vi "首页.vi"() -> ()   [LabVIEW 2016]
uses:
  <vilib>/Utility/miscctls.llb/LVPointTypeDef.ctl
  <vilib>/addons/database/_DB Variant To Data/Database Variant To Data.xnode
  PLC/PLC.lvlib
panel:
  out "大项目框 12":T1(xcontrol)
  out "大项目框 11":T1(xcontrol)
  out "大项目框 10":T1(xcontrol)
  out "大项目框 9":T1(xcontrol)
  out "大项目框 8":T1(xcontrol)
  out "大项目框 7":T1(xcontrol)
  out "大项目框 6":T1(xcontrol)
  out "大项目框 5":T1(xcontrol)
  out "大项目框 4":T1(xcontrol)
  out "大项目框 3":T1(xcontrol)
  out "大项目框 2":T1(xcontrol)
  out "大项目框":T1(xcontrol)
  out "湿度":string="75.5 %"
  out "室温":string="25.8 ℃"
  # "室温:"
  # "湿度:"
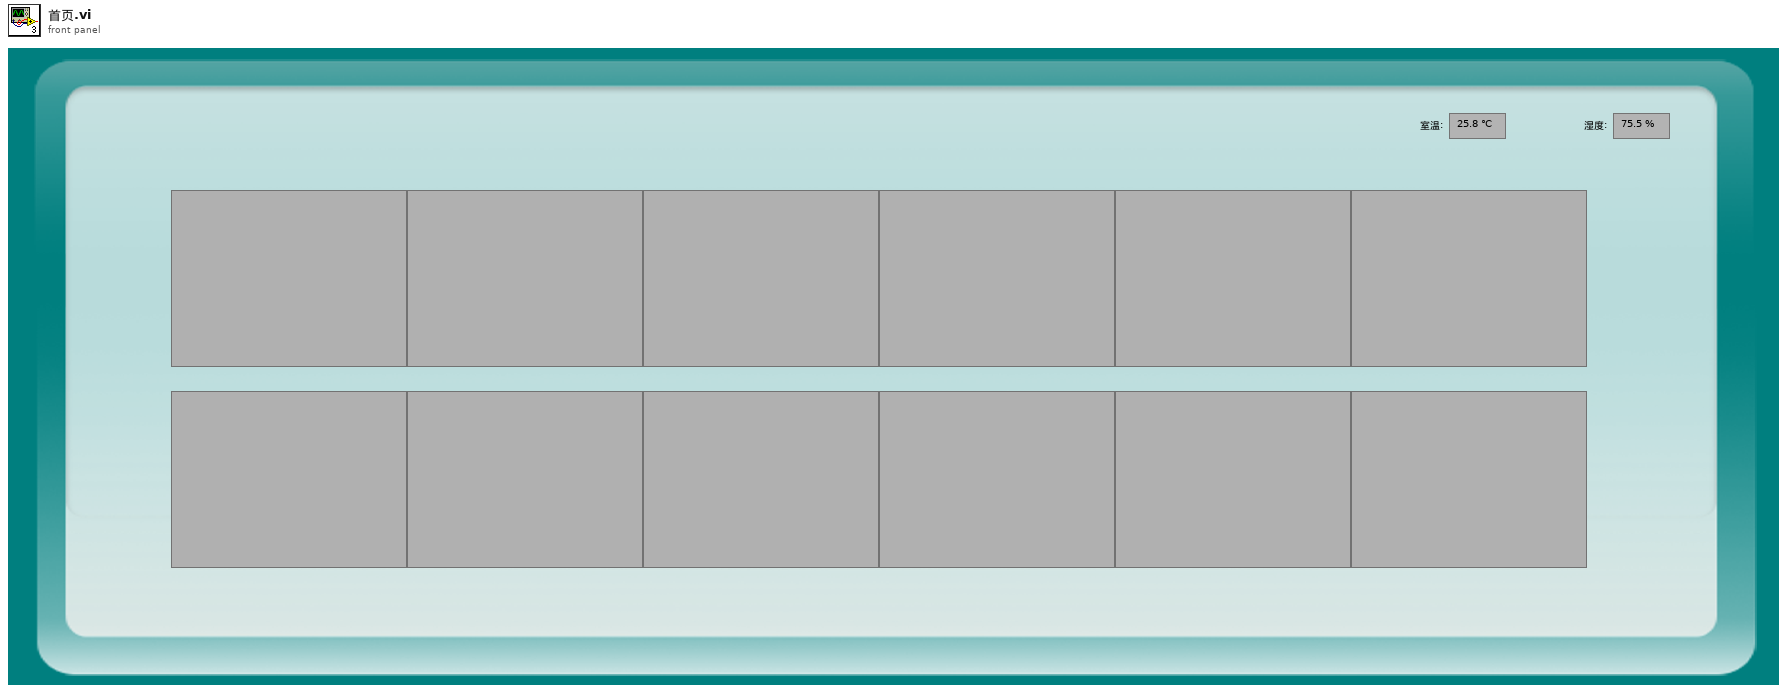
[diagram p1: front panel]
types:
  T1 = cluster{"中文项目名称":string, "英文项目名称":string, "单位":string, "浓度值":string}
  T2 = typedef "LVPointTypeDef.ctl" = cluster{"Horizontal":i16, "Vertical":i16}
  T3 = cluster{"显示参数中文名":string, "显示参数英文名":string, "显示浓度":string, "显示单位":string}[]
  T4 = cluster{"显示参数中文名":string, "显示参数英文名":string, "显示浓度":string, "显示单位":string}
  T5 = cluster{"AD0":sgl, "AD1":sgl, "AD2":sgl, "AD3":sgl, "AD4":sgl, "AD5":sgl}
  T6 = typedef "LVDateTimeRec.ctl" = cluster{"秒数的小数部分":dbl, "秒":i32, "分":i32, "时":i32, "日":i32, "月":i32, "年":i32, "天数（周）":i32, "天数（年）":i32, "DST":i32}
  T7 = cluster{"时间标识":timestamp, "监测值":sgl, "单位":string}
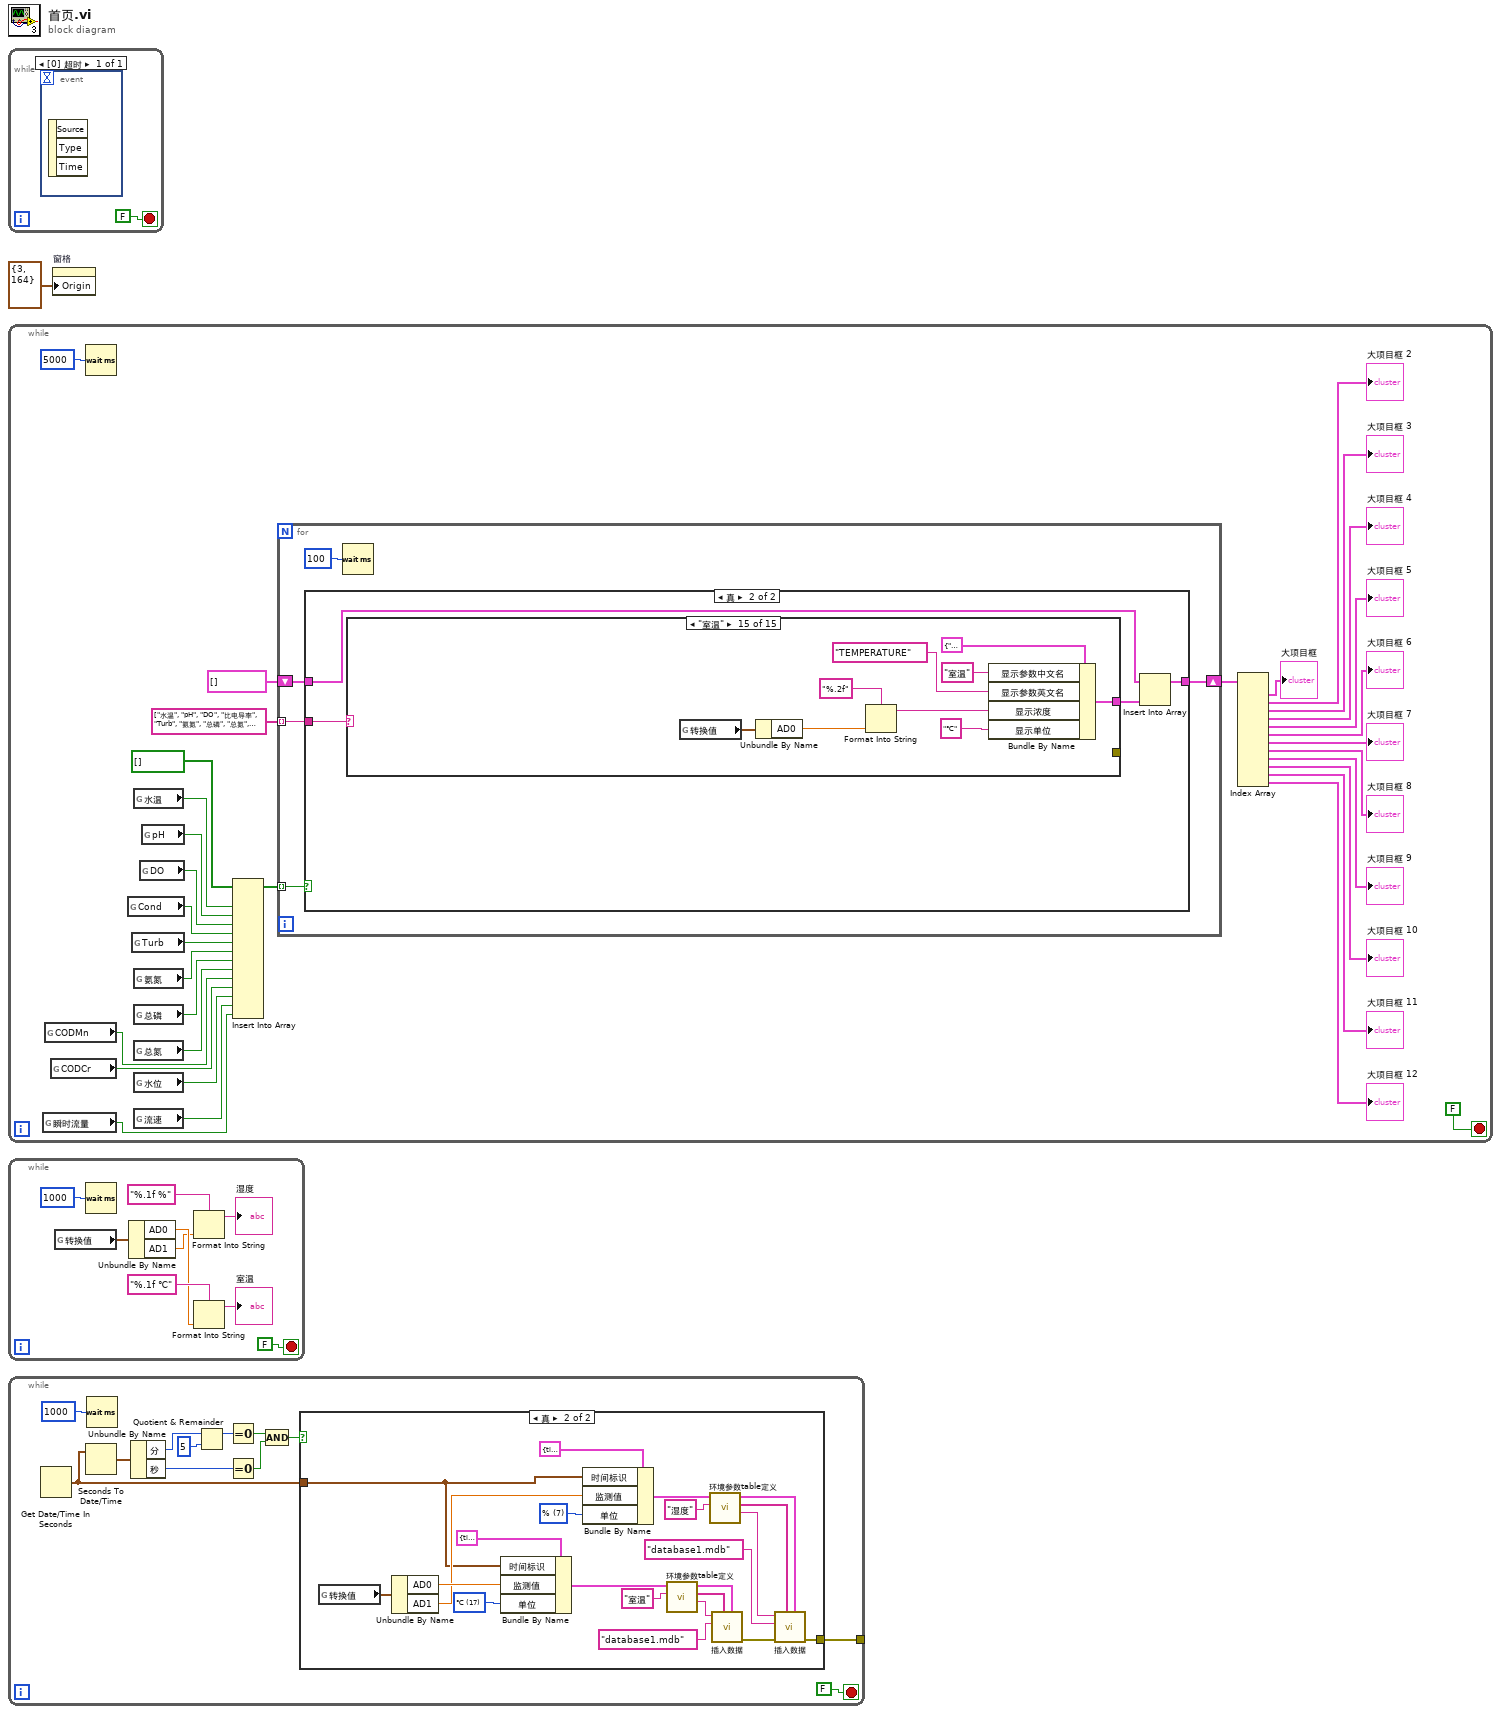
[diagram p0: block diagram]
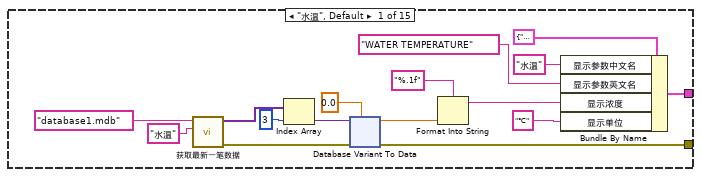
[diagram p4: hidden frame]
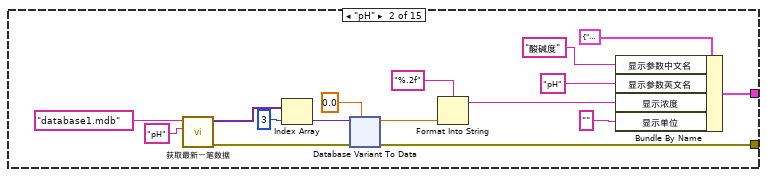
[diagram p5: hidden frame]
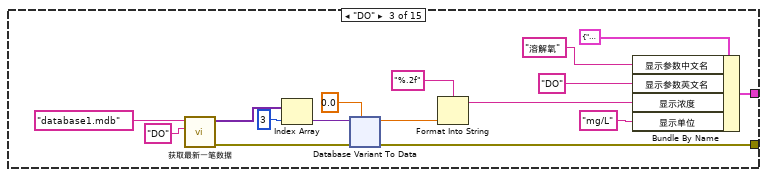
[diagram p6: hidden frame]
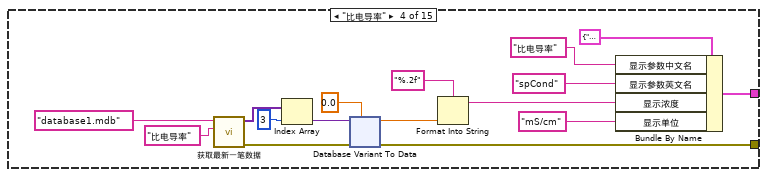
[diagram p7: hidden frame]
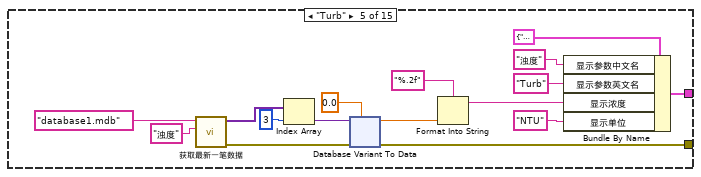
[diagram p8: hidden frame]
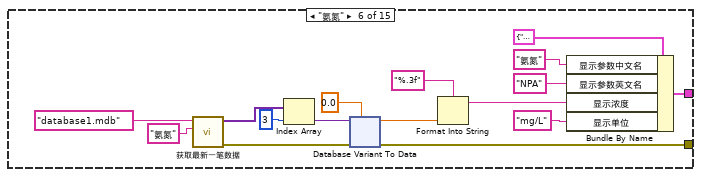
[diagram p9: hidden frame]
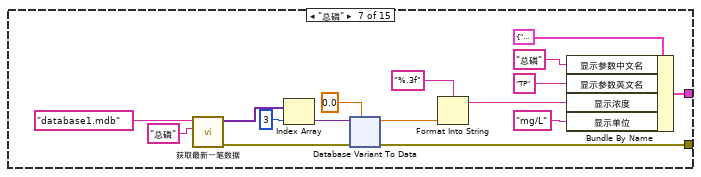
[diagram p10: hidden frame]
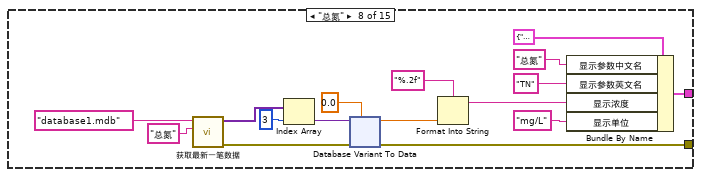
[diagram p11: hidden frame]
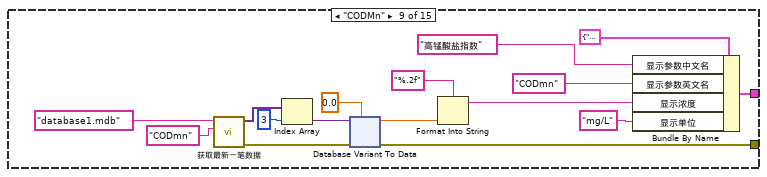
[diagram p12: hidden frame]
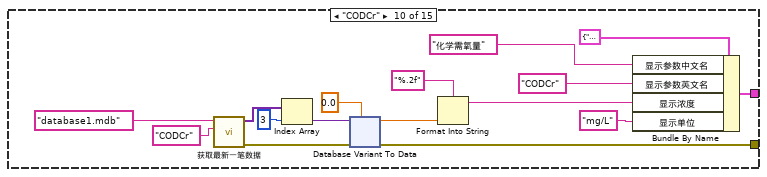
[diagram p13: hidden frame]
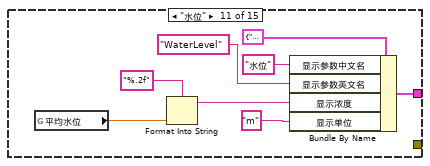
[diagram p14: hidden frame]
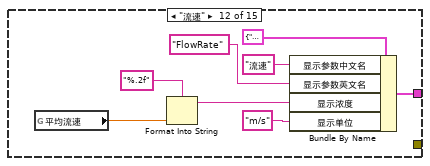
[diagram p15: hidden frame]
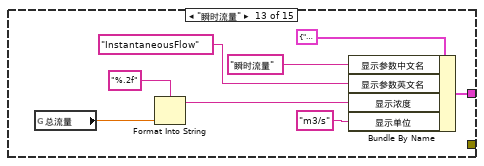
[diagram p16: hidden frame]
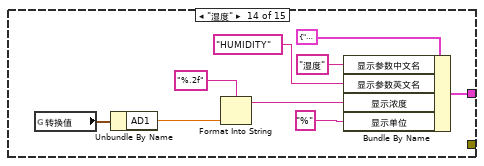
[diagram p17: hidden frame]
diagram:
  n1 = while {
    stop <- FALSE stop-if-true
    n2 = event shown="[0] 超时" {
      selector: _ -> [_]
      dyn-events: _ -> [_]
      timeout: _ -> [_]
      event Timeout {
        n3 = event-data() -> ()  [unwired: 1 in, 3 out]
      }
    }
  }
  n4 = while {
    stop <- FALSE stop-if-true
    n5 = global read "副屏设置全局变量.vi" "瞬时流量"() -> (w30:bool)
    n6 = global read "副屏设置全局变量.vi" "CODMn"() -> (w26:bool)
    n7 = global read "副屏设置全局变量.vi" "CODCr"() -> (w27:bool)
    n8 = Wait (ms)(milliseconds to wait=u32 5000 ("等待时间（毫秒）")) -> ()  [unwired: 1 out]
    n9 = global read "副屏设置全局变量.vi" "Cond"() -> (w21:bool)
    n10 = global read "副屏设置全局变量.vi" "Turb"() -> (w22:bool)
    n11 = global read "副屏设置全局变量.vi" "水温"() -> (w18:bool)
    n12 = global read "副屏设置全局变量.vi" "氨氮"() -> (w23:bool)
    n13 = global read "副屏设置全局变量.vi" "总磷"() -> (w24:bool)
    n14 = global read "副屏设置全局变量.vi" "总氮"() -> (w25:bool)
    n15 = global read "副屏设置全局变量.vi" "水位"() -> (w28:bool)
    n16 = global read "副屏设置全局变量.vi" "流速"() -> (w29:bool)
    n17 = global read "副屏设置全局变量.vi" "DO"() -> (w20:bool)
    n18 = global read "副屏设置全局变量.vi" "pH"() -> (w19:bool)
    n19 = Insert Into Array(array=bool[] [], new element #1=w18, new element #2=w19, new element #3=w20, new element #4=w21, new element #5=w22, new element #6=w23, new element #7=w24, new element #8=w25, new element #9=w26, new element #10=w27, new element #11=w28, new element #12=w29, new element #13=w30) -> (w32:bool[])  [unwired: 1 in]
    n20 = for {
      tunnel: w32 -> [w39] mode=indexing
      tunnel: string[] ["水温", "pH", "DO", "比电导率", "Turb", "氨氮", "总磷", "总氮", "CODMn", "CODCr", "水位", "流速", "瞬时流量"] -> [w38] mode=indexing
      shift-right: [w36] -> w16
      shift-left: T3 [] -> [w37]
      n21 = case shown="真" w39 {
        tunnel: w38 -> [_ w44]
        tunnel: w37 -> [w40 w43]
        tunnel: [w40 w42] -> w36
        frame False {
        }
        frame True {
          n22 = case shown="\"室温\"" w44 {
            tunnel: [w45 w104 w152 w200 w248 w296 w344 w392 w440 w488 w528 w536 w541 w553 w562] -> w41
            tunnel: [w46 w93 w141 w189 w237 w285 w333 w381 w429 w477 _ _ _ _ _] -> _
            frame "水温", Default {
              n23 = call "获取最新一笔数据.vi"("table"="水温", "database"="database1.mdb" ("名称或相对路径")) -> ("error out"=w47:errorcluster, "子数组"=w53:variant[])  [unwired: 8 in]
              n24 = Index Array(array=w53, index=3 ("索引")) -> (element=w51:variant)
              n25 = xnode "Database Variant To Data"("database variant"=w51, "error in (no error)"=w47, "type"=0.0) -> ("data"=w48:dbl, "error out"=w46:errorcluster)
              n26 = Format Into String(format string="%.1f" ("格式字符串"), w48) -> (resulting string=w55:string)  [unwired: 2 in, 1 out]
              n27 = Bundle By Name(cluster=T4 {"显示参数中文名"="", "显示参数英文名"="", "显示浓度"="", "显示单位"=""} ("元素"), "显示参数中文名"="水温", "显示参数英文名"="WATER TEMPERATURE", "显示浓度"=w55, "显示单位"="℃") -> (w45:T4)
            }
            frame "pH" {
              n28 = call "获取最新一笔数据.vi"("table"="pH", "database"="database1.mdb" ("名称或相对路径")) -> ("error out"=w94:errorcluster, "子数组"=w100:variant[])  [unwired: 8 in]
              n29 = Index Array(array=w100, index=3 ("索引")) -> (element=w98:variant)
              n30 = xnode "Database Variant To Data"("database variant"=w98, "error in (no error)"=w94, "type"=0.0) -> ("data"=w95:dbl, "error out"=w93:errorcluster)
              n31 = Format Into String(format string="%.2f" ("格式字符串"), w95) -> (resulting string=w102:string)  [unwired: 2 in, 1 out]
              n32 = Bundle By Name(cluster=T4 {"显示参数中文名"="", "显示参数英文名"="", "显示浓度"="", "显示单位"=""} ("元素"), "显示参数中文名"="酸碱度", "显示参数英文名"="pH", "显示浓度"=w102, "显示单位"="") -> (w104:T4)
            }
            frame "DO" {
              n33 = call "获取最新一笔数据.vi"("table"="DO", "database"="database1.mdb" ("名称或相对路径")) -> ("error out"=w142:errorcluster, "子数组"=w148:variant[])  [unwired: 8 in]
              n34 = Index Array(array=w148, index=3 ("索引")) -> (element=w146:variant)
              n35 = xnode "Database Variant To Data"("database variant"=w146, "error in (no error)"=w142, "type"=0.0) -> ("data"=w143:dbl, "error out"=w141:errorcluster)
              n36 = Format Into String(format string="%.2f" ("格式字符串"), w143) -> (resulting string=w150:string)  [unwired: 2 in, 1 out]
              n37 = Bundle By Name(cluster=T4 {"显示参数中文名"="", "显示参数英文名"="", "显示浓度"="", "显示单位"=""} ("元素"), "显示参数中文名"="溶解氧", "显示参数英文名"="DO", "显示浓度"=w150, "显示单位"="mg/L") -> (w152:T4)
            }
            frame "比电导率" {
              n38 = call "获取最新一笔数据.vi"("table"="比电导率", "database"="database1.mdb" ("名称或相对路径")) -> ("error out"=w190:errorcluster, "子数组"=w196:variant[])  [unwired: 8 in]
              n39 = Index Array(array=w196, index=3 ("索引")) -> (element=w194:variant)
              n40 = xnode "Database Variant To Data"("database variant"=w194, "error in (no error)"=w190, "type"=0.0) -> ("data"=w191:dbl, "error out"=w189:errorcluster)
              n41 = Format Into String(format string="%.2f" ("格式字符串"), w191) -> (resulting string=w198:string)  [unwired: 2 in, 1 out]
              n42 = Bundle By Name(cluster=T4 {"显示参数中文名"="", "显示参数英文名"="", "显示浓度"="", "显示单位"=""} ("元素"), "显示参数中文名"="比电导率", "显示参数英文名"="spCond", "显示浓度"=w198, "显示单位"="mS/cm") -> (w200:T4)
            }
            frame "Turb" {
              n43 = call "获取最新一笔数据.vi"("table"="浊度", "database"="database1.mdb" ("名称或相对路径")) -> ("error out"=w238:errorcluster, "子数组"=w244:variant[])  [unwired: 8 in]
              n44 = Index Array(array=w244, index=3 ("索引")) -> (element=w242:variant)
              n45 = xnode "Database Variant To Data"("database variant"=w242, "error in (no error)"=w238, "type"=0.0) -> ("data"=w239:dbl, "error out"=w237:errorcluster)
              n46 = Format Into String(format string="%.2f" ("格式字符串"), w239) -> (resulting string=w246:string)  [unwired: 2 in, 1 out]
              n47 = Bundle By Name(cluster=T4 {"显示参数中文名"="", "显示参数英文名"="", "显示浓度"="", "显示单位"=""} ("元素"), "显示参数中文名"="浊度", "显示参数英文名"="Turb", "显示浓度"=w246, "显示单位"="NTU") -> (w248:T4)
            }
            frame "氨氮" {
              n48 = call "获取最新一笔数据.vi"("table"="氨氮", "database"="database1.mdb" ("名称或相对路径")) -> ("error out"=w286:errorcluster, "子数组"=w292:variant[])  [unwired: 8 in]
              n49 = Index Array(array=w292, index=3 ("索引")) -> (element=w290:variant)
              n50 = xnode "Database Variant To Data"("database variant"=w290, "error in (no error)"=w286, "type"=0.0) -> ("data"=w287:dbl, "error out"=w285:errorcluster)
              n51 = Format Into String(format string="%.3f" ("格式字符串"), w287) -> (resulting string=w294:string)  [unwired: 2 in, 1 out]
              n52 = Bundle By Name(cluster=T4 {"显示参数中文名"="", "显示参数英文名"="", "显示浓度"="", "显示单位"=""} ("元素"), "显示参数中文名"="氨氮", "显示参数英文名"="NPA", "显示浓度"=w294, "显示单位"="mg/L") -> (w296:T4)
            }
            frame "总磷" {
              n53 = call "获取最新一笔数据.vi"("table"="总磷", "database"="database1.mdb" ("名称或相对路径")) -> ("error out"=w334:errorcluster, "子数组"=w340:variant[])  [unwired: 8 in]
              n54 = Index Array(array=w340, index=3 ("索引")) -> (element=w338:variant)
              n55 = xnode "Database Variant To Data"("database variant"=w338, "error in (no error)"=w334, "type"=0.0) -> ("data"=w335:dbl, "error out"=w333:errorcluster)
              n56 = Format Into String(format string="%.3f" ("格式字符串"), w335) -> (resulting string=w342:string)  [unwired: 2 in, 1 out]
              n57 = Bundle By Name(cluster=T4 {"显示参数中文名"="", "显示参数英文名"="", "显示浓度"="", "显示单位"=""} ("元素"), "显示参数中文名"="总磷", "显示参数英文名"="TP", "显示浓度"=w342, "显示单位"="mg/L") -> (w344:T4)
            }
            frame "总氮" {
              n58 = call "获取最新一笔数据.vi"("table"="总氮", "database"="database1.mdb" ("名称或相对路径")) -> ("error out"=w382:errorcluster, "子数组"=w388:variant[])  [unwired: 8 in]
              n59 = Index Array(array=w388, index=3 ("索引")) -> (element=w386:variant)
              n60 = xnode "Database Variant To Data"("database variant"=w386, "error in (no error)"=w382, "type"=0.0) -> ("data"=w383:dbl, "error out"=w381:errorcluster)
              n61 = Format Into String(format string="%.2f" ("格式字符串"), w383) -> (resulting string=w390:string)  [unwired: 2 in, 1 out]
              n62 = Bundle By Name(cluster=T4 {"显示参数中文名"="", "显示参数英文名"="", "显示浓度"="", "显示单位"=""} ("元素"), "显示参数中文名"="总氮", "显示参数英文名"="TN", "显示浓度"=w390, "显示单位"="mg/L") -> (w392:T4)
            }
            frame "CODMn" {
              n63 = call "获取最新一笔数据.vi"("table"="CODmn", "database"="database1.mdb" ("名称或相对路径")) -> ("error out"=w430:errorcluster, "子数组"=w436:variant[])  [unwired: 8 in]
              n64 = Index Array(array=w436, index=3 ("索引")) -> (element=w434:variant)
              n65 = xnode "Database Variant To Data"("database variant"=w434, "error in (no error)"=w430, "type"=0.0) -> ("data"=w431:dbl, "error out"=w429:errorcluster)
              n66 = Format Into String(format string="%.2f" ("格式字符串"), w431) -> (resulting string=w438:string)  [unwired: 2 in, 1 out]
              n67 = Bundle By Name(cluster=T4 {"显示参数中文名"="", "显示参数英文名"="", "显示浓度"="", "显示单位"=""} ("元素"), "显示参数中文名"="高锰酸盐指数", "显示参数英文名"="CODmn", "显示浓度"=w438, "显示单位"="mg/L") -> (w440:T4)
            }
            frame "CODCr" {
              n68 = call "获取最新一笔数据.vi"("table"="CODCr", "database"="database1.mdb" ("名称或相对路径")) -> ("error out"=w478:errorcluster, "子数组"=w484:variant[])  [unwired: 8 in]
              n69 = Index Array(array=w484, index=3 ("索引")) -> (element=w482:variant)
              n70 = xnode "Database Variant To Data"("database variant"=w482, "error in (no error)"=w478, "type"=0.0) -> ("data"=w479:dbl, "error out"=w477:errorcluster)
              n71 = Format Into String(format string="%.2f" ("格式字符串"), w479) -> (resulting string=w486:string)  [unwired: 2 in, 1 out]
              n72 = Bundle By Name(cluster=T4 {"显示参数中文名"="", "显示参数英文名"="", "显示浓度"="", "显示单位"=""} ("元素"), "显示参数中文名"="化学需氧量", "显示参数英文名"="CODCr", "显示浓度"=w486, "显示单位"="mg/L") -> (w488:T4)
            }
            frame "水位" {
              n73 = global read "流量计全局变量.vi" "平均水位"() -> (w525:dbl)
              n74 = Format Into String(format string="%.2f" ("格式字符串"), w525) -> (resulting string=w526:string)  [unwired: 2 in, 1 out]
              n75 = Bundle By Name(cluster=T4 {"显示参数中文名"="", "显示参数英文名"="", "显示浓度"="", "显示单位"=""} ("元素"), "显示参数中文名"="水位", "显示参数英文名"="WaterLevel", "显示浓度"=w526, "显示单位"="m") -> (w528:T4)
            }
            frame "流速" {
              n76 = global read "流量计全局变量.vi" "平均流速"() -> (w533:dbl)
              n77 = Format Into String(format string="%.2f" ("格式字符串"), w533) -> (resulting string=w534:string)  [unwired: 2 in, 1 out]
              n78 = Bundle By Name(cluster=T4 {"显示参数中文名"="", "显示参数英文名"="", "显示浓度"="", "显示单位"=""} ("元素"), "显示参数中文名"="流速", "显示参数英文名"="FlowRate", "显示浓度"=w534, "显示单位"="m/s") -> (w536:T4)
            }
            frame "瞬时流量" {
              n79 = global read "流量计全局变量.vi" "总流量"() -> (w542:dbl)
              n80 = Format Into String(format string="%.2f" ("格式字符串"), w542) -> (resulting string=w543:string)  [unwired: 2 in, 1 out]
              n81 = Bundle By Name(cluster=T4 {"显示参数中文名"="", "显示参数英文名"="", "显示浓度"="", "显示单位"=""} ("元素"), "显示参数中文名"="瞬时流量", "显示参数英文名"="InstantaneousFlow", "显示浓度"=w543, "显示单位"="m3/s") -> (w541:T4)
            }
            frame "湿度" {
              n82 = global read "采配水全局变量.vi" "转换值"() -> (w550:T5)
              n83 = Unbundle By Name(w550) -> ("AD1"=w552:sgl)
              n84 = Format Into String(format string="%.2f" ("格式字符串"), w552) -> (resulting string=w549:string)  [unwired: 2 in, 1 out]
              n85 = Bundle By Name(cluster=T4 {"显示参数中文名"="", "显示参数英文名"="", "显示浓度"="", "显示单位"=""} ("元素"), "显示参数中文名"="湿度", "显示参数英文名"="HUMIDITY", "显示浓度"=w549, "显示单位"="%") -> (w553:T4)
            }
            frame "室温" {
              n86 = global read "采配水全局变量.vi" "转换值"() -> (w559:T5)
              n87 = Unbundle By Name(w559) -> ("AD0"=w561:sgl)
              n88 = Format Into String(format string="%.2f" ("格式字符串"), w561) -> (resulting string=w558:string)  [unwired: 2 in, 1 out]
              n89 = Bundle By Name(cluster=T4 {"显示参数中文名"="", "显示参数英文名"="", "显示浓度"="", "显示单位"=""} ("元素"), "显示参数中文名"="室温", "显示参数英文名"="TEMPERATURE", "显示浓度"=w558, "显示单位"="℃") -> (w562:T4)
            }
          }
          n90 = Insert Into Array(array=w43, new element=w41) -> (w42:T3)  [unwired: 1 in]
        }
      }
      n91 = Wait (ms)(milliseconds to wait=u32 100 ("等待时间（毫秒）")) -> ()  [unwired: 1 out]
    }
    n92 = Index Array(array=w16) -> (element #1=→"大项目框":T4, element #2=→"大项目框 2":T4, element #3=→"大项目框 3":T4, element #4=→"大项目框 4":T4, element #5=→"大项目框 5":T4, element #6=→"大项目框 6":T4, element #7=→"大项目框 7":T4, element #8=→"大项目框 8":T4, element #9=→"大项目框 9":T4, element #10=→"大项目框 10":T4, element #11=→"大项目框 11":T4, element #12=→"大项目框 12":T4)  [unwired: 12 in]
  }
  n93 = while {
    stop <- FALSE stop-if-true
    n94 = global read "采配水全局变量.vi" "转换值"() -> (w573:T5)
    n95 = Wait (ms)(milliseconds to wait=u32 1000 ("等待时间（毫秒）")) -> ()  [unwired: 1 out]
    n96 = Unbundle By Name(w573) -> ("AD0"=w568:sgl, "AD1"=w567:sgl)
    n97 = Format Into String(format string="%.1f %" ("格式字符串"), w567) -> (resulting string=→"湿度":string)  [unwired: 2 in, 1 out]
    n98 = Format Into String(format string="%.1f ℃" ("格式字符串"), w568) -> (resulting string=→"室温":string)  [unwired: 2 in, 1 out]
  }
  n99 = while {
    tunnel: [w586] -> _
    stop <- FALSE stop-if-true
    n100 = Get Date/Time In Seconds() -> (seconds since 1Jan1904=w585:timestamp)
    n101 = Seconds To Date/Time(time stamp (now)=w585) -> (date time rec=w584:T6)  [unwired: 1 in]
    n102 = Wait (ms)(milliseconds to wait=u32 1000 ("等待时间（毫秒）")) -> ()  [unwired: 1 out]
    n103 = Unbundle By Name(w584) -> ("分"=w583:i32, "秒"=w581:i32)
    n104 = Quotient & Remainder(x=w583, y=5) -> (x-y*floor(x/y)=w580:i32)  [unwired: 1 out]
    n105 = Equal To 0?(x=w580) -> (x = 0?=w579:bool)
    n106 = Equal To 0?(x=w581) -> (x = 0?=w578:bool)
    n107 = Compound Arithmetic op=AND ("复合运算")(w579, w578) -> (w577:bool)
    n108 = case shown="真" w577 {
      tunnel: [_ w601] -> w586
      tunnel: w585 -> [_ w589]
      frame False {
      }
      frame True {
        w594 = u16 7 items=["ug/L", "mg/L", "ppm", "mg/m3", "cm", "ppb", "ug/m3", "%", "nmol/mol", "umol/mol", "MPN/L", "MPN/100ml", "ng/m3", "NTU", "无量纲", "ms/cm", "us/cm", "℃", "V"] ("单位")
        w598 = u16 17 items=["ug/L", "mg/L", "ppm", "mg/m3", "cm", "ppb", "ug/m3", "%", "nmol/mol", "umol/mol", "MPN/L", "MPN/100ml", "ng/m3", "NTU", "无量纲", "ms/cm", "us/cm", "℃", "V"] ("单位")
        n109 = global read "采配水全局变量.vi" "转换值"() -> (w609:T5)
        n110 = Unbundle By Name(w609) -> ("AD0"=w597:sgl, "AD1"=w595:sgl)
        n111 = Bundle By Name(cluster=cluster{"时间标识":timestamp, "监测值":sgl, "单位":u16} {"时间标识"=timestamp(0 s since 1904-01-01), "监测值"=0.0, "单位"=0} ("data"), "时间标识"=w589, "监测值"=w597, "单位"=w598) -> (w599:cluster{"时间标识":timestamp, "监测值":sgl, "单位":u16})
        n112 = Bundle By Name(cluster=cluster{"时间标识":timestamp, "监测值":sgl, "单位":u16} {"时间标识"=timestamp(0 s since 1904-01-01), "监测值"=0.0, "单位"=0} ("data"), "时间标识"=w589, "监测值"=w595, "单位"=w594) -> (w593:cluster{"时间标识":timestamp, "监测值":sgl, "单位":u16})
        n113 = call "环境参数table定义.vi"("table 输入"="室温", "data"=w599) -> ("table 输出"=w608:string, "columns"=w607:string[], "data输出"=w606:T7)  [unwired: 7 in]
        n114 = call "环境参数table定义.vi"("table 输入"="湿度", "data"=w593) -> ("table 输出"=w603:string, "columns"=w604:string[], "data输出"=w605:T7)  [unwired: 7 in]
        n115 = call "插入数据.vi"("data"=w606, "columns"=w607, "database"="database1.mdb" ("table 输入"), "table"=w608) -> ("error out"=w602:errorcluster)  [unwired: 7 in]
        n116 = call "插入数据.vi"("data"=w605, "columns"=w604, "error in (no error)"=w602, "database"="database1.mdb" ("table 输入"), "table"=w603) -> ("error out"=w601:errorcluster)  [unwired: 6 in]
      }
    }
  }
  n117 = property on="窗格" class="Pane"("Origin"=T2 {"Horizontal"=3, "Vertical"=164} ("原点")) -> ()  [unwired: 2 in, 2 out]
